vi "Reset Strafe Encoder.vi"   [LabVIEW 2014]
types:
  T1 = typedef "WPI_EncoderDevRef.ctl" = cluster{"DevStatus":errorcluster, "EncoderIndex":T2, "CounterIndex":T3, "DistancePerCount":dbl, "Decoding Type":T4}
  T2 = typedef "FPGA_EncoderIdx.ctl" = enum8{"Enc 0", "Enc 1", "Enc 2", "Enc 3", "Enc 4", "Enc 5", "Enc 6", "Enc 7", "Invalid"}
  T3 = typedef "FPGA_CounterCtrSystemIndex.ctl" = enum8{"Ctr 0", "Ctr 1", "Ctr 2", "Ctr 3", "Ctr 4", "Ctr 5", "Ctr 6", "Ctr 7", "Invalid"}
  T4 = typedef "WPI_EncoderType.ctl" = enum16{"1x", "2x", "4x"}
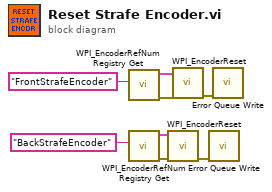
[diagram p0: block diagram]
diagram:
  n1 = call <vilib>:"WPI_EncoderRefNum Registry Get.vi"("refnum name"="FrontStrafeEncoder") -> ("error out"=w3:errorcluster, "EncoderDevRef"=w4:T1)  [unwired: 9 in]
  n2 = call <vilib>:"WPI_EncoderRefNum Registry Get.vi"("refnum name"="BackStrafeEncoder") -> ("error out"=w5:errorcluster, "EncoderDevRef"=w6:T1)  [unwired: 9 in]
  n3 = call <vilib>:"WPI_EncoderReset.vi"("error in (no error)"=w5, "EncoderDevRef"=w6) -> ("error out"=w8:errorcluster)  [unwired: 8 in, 1 out]
  n4 = call <vilib>:"WPI_EncoderReset.vi"("error in (no error)"=w3, "EncoderDevRef"=w4) -> ("error out"=w7:errorcluster)  [unwired: 8 in, 1 out]
  n5 = call "Error Queue Write.vi"("error in (no error)"=w8) -> ()  [unwired: 11 in]
  n6 = call "Error Queue Write.vi"("error in (no error)"=w7) -> ()  [unwired: 11 in]
